vi "UpdateMeasurementTestElement.vi"(0 "TestSeqClass in":refnum<class "TestSeqClass.lvclass">, 5 "TestMeasureStep.lvclass":refnum<class "TestMeasureStep.lvclass">, 11 "error in (no error)":errorcluster) -> (4 "TestSeqClass out":refnum<class "TestSeqClass.lvclass">, 15 "error out":errorcluster)   [LabVIEW 2017]
uses:
  TestSeqClass.lvclass
  TestMeasureStep/TestMeasureStep.lvclass
  TestSeqClass.lvclass/TestSeqClass.ctl
  Read CurrentTestPointer.vi
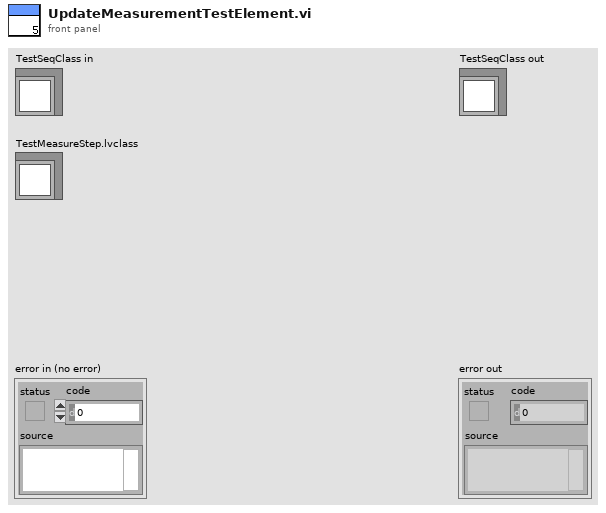
[diagram p1: front panel]
types:
  T1 = typedef "TestSeqType.ctl" = refnum<class "TestMeasureStep.lvclass">[]
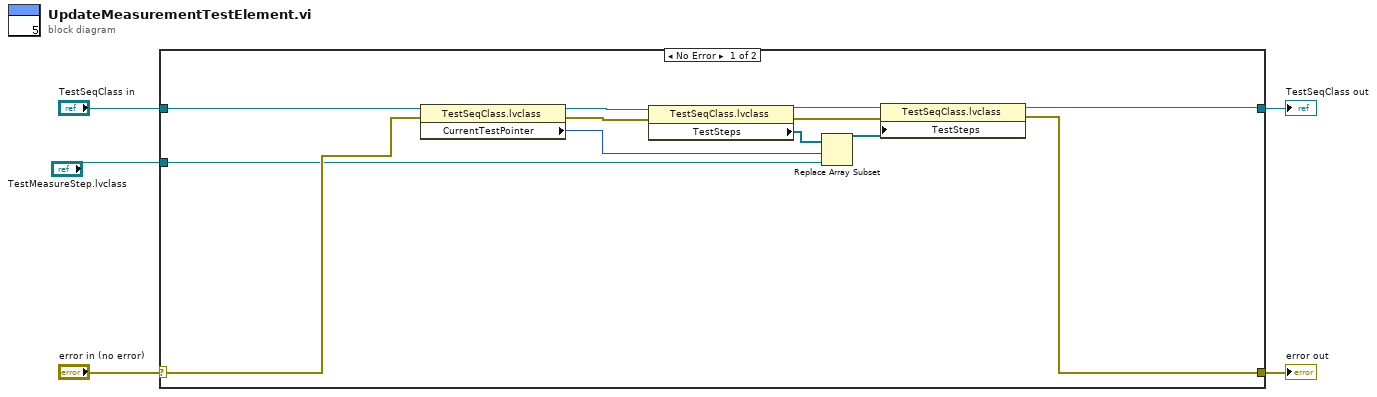
[diagram p0: block diagram]
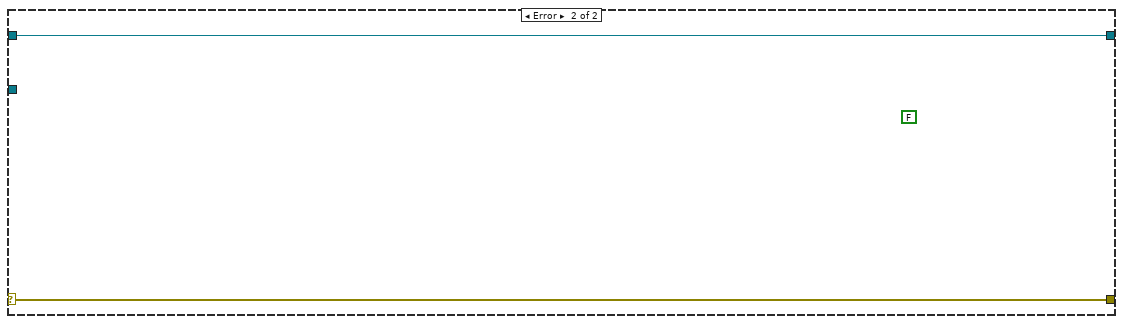
[diagram p2: hidden frame]
diagram:
  n1 = case shown="No Error" "error in (no error)" {
    selector: "error in (no error)" -> [w16 w19]
    tunnel: [w6 w19] -> w4
    tunnel: [w7 w18] -> w2
    tunnel: "TestSeqClass in" -> [w17 w18]
    tunnel: "TestMeasureStep.lvclass" -> [w12 _]
    frame No Error {
      n2 = property class="TestSeqClass.lvclass"(reference=w17, error in=w16) -> (reference out=w15:refnum<class "TestSeqClass.lvclass">, error out=w14:errorcluster, "CurrentTestPointer"=w11:u32)
      n3 = property class="TestSeqClass.lvclass"(reference=w15, error in=w14) -> (reference out=w9:refnum<class "TestSeqClass.lvclass">, error out=w8:errorcluster, "TestSteps"=w13:T1)
      n4 = Replace Array Subset(array=w13, new element=w12, index=w11) -> (w10:T1)
      n5 = property class="TestSeqClass.lvclass"(reference=w9, error in=w8, "TestSteps"=w10) -> (reference out=w7:refnum<class "TestSeqClass.lvclass">, error out=w6:errorcluster)
    }
    frame Error {
      (unwired) FALSE
    }
  }
  "error out" <- w4
  "TestSeqClass out" <- w2
